vi "FRIC_navX_Internal_Serial_GenerateCommand.vi"(11 "I2C Process Loop TypeDef (in)":T1={"State Array"=[enum."INI", enum."Open"], "error"={"status"=FALSE, "code"=0, "source"=""}, "FPGA Cluster"={"Last Valid FPGA Time"=0.0, "Error Count"=0, "Initialized"=FALSE}, "Device Info"={"Interface"={"Protocol"=enum."SERIAL", "Update Rate (4Hz-100Hz)"=4, "navX Open TypeDef"=variant}, "Notify Packet"=refnum, "Loop VI Refnum"=refnum, "Ready to Close Occurrence Refnum"=refnum, "Name"=""}, "I2CDevRef"={"DevStatus"={"status"=FALSE, "code"=0, "source"=""}, "Controller"=enum."Controller 1", "Device Address"=0, "Handle"=0, "I2C Bus"=enum."Invalid"}, "Registry"=[], "Command Array"=[214, 32], "Connected?"=FALSE, "navX Device Memory Size"=85, "notification"={"navX Action"=enum."None", "Data"=variant}, "Memory Size Set"=FALSE, "SPIDevRef"={"DevStatus"={"status"=FALSE, "code"=0, "source"=""}, "Handle"=0, "Controller"=enum."Controller 1", "SPI Bus"=enum."SPI On-Board, CS0"}, "navX Serial Open"={"Serial Port"=enum."Onboard RS-232", "Stream Type"=enum."YRPH"}, "SerialPortRef"={"DevStatus"={"status"=FALSE, "code"=0, "source"=""}, "Serial Port Name"=""}, "Serial Read Buffer"="", "Serial Write Buffer"=[], "Device Number"=enum."Dev0"} {"navX Device Memory Size" format="%x"; "Command Array" items=["UNDEFINED"=0, "NAVX_INTEGRATION_CTL_RESET_VEL_X"=1, "NAVX_INTEGRATION_CTL_RESET_VEL_Y"=2, "NAVX_INTEGRATION_CTL_RESET_VEL_Z"=4, "NAVX_INTEGRATION_CTL_RESET_DISP_X"=8, "NAVX_INTEGRATION_CTL_RESET_DISP_Y"=16, "NAVX_INTEGRATION_CTL_RESET_DISP_Z"=32, "NAVX_INTEGRATION_CTL_RESET_YAW"=128]; "I2CDevRef"."Device Address" format="%.0x"; "Device Info"."Interface"."Update Rate (4Hz-100Hz)" min=4 max=60 step=1}) -> (3 "I2C Process Loop TypeDef (out)":T1={"State Array"=[enum."INI", enum."Open"], "error"={"status"=FALSE, "code"=0, "source"=""}, "FPGA Cluster"={"Last Valid FPGA Time"=0.0, "Error Count"=0, "Initialized"=FALSE}, "Device Info"={"Interface"={"Protocol"=enum."SERIAL", "Update Rate (4Hz-100Hz)"=4, "navX Open TypeDef"=variant}, "Notify Packet"=refnum, "Loop VI Refnum"=refnum, "Ready to Close Occurrence Refnum"=refnum, "Name"=""}, "I2CDevRef"={"DevStatus"={"status"=FALSE, "code"=0, "source"=""}, "Controller"=enum."Controller 1", "Device Address"=0, "Handle"=0, "I2C Bus"=enum."Invalid"}, "Registry"=[], "Command Array"=[], "Connected?"=FALSE, "navX Device Memory Size"=85, "notification"={"navX Action"=enum."None", "Data"=variant}, "Memory Size Set"=FALSE, "SPIDevRef"={"DevStatus"={"status"=FALSE, "code"=0, "source"=""}, "Handle"=0, "Controller"=enum."Controller 1", "SPI Bus"=enum."SPI On-Board, CS0"}, "navX Serial Open"={"Serial Port"=enum."Onboard RS-232", "Stream Type"=enum."YRPH"}, "SerialPortRef"={"DevStatus"={"status"=FALSE, "code"=0, "source"=""}, "Serial Port Name"=""}, "Serial Read Buffer"="", "Serial Write Buffer"=[], "Device Number"=enum."Dev0"} {"navX Device Memory Size" format="%x"; "Command Array" items=["UNDEFINED"=0, "NAVX_INTEGRATION_CTL_RESET_VEL_X"=1, "NAVX_INTEGRATION_CTL_RESET_VEL_Y"=2, "NAVX_INTEGRATION_CTL_RESET_VEL_Z"=4, "NAVX_INTEGRATION_CTL_RESET_DISP_X"=8, "NAVX_INTEGRATION_CTL_RESET_DISP_Y"=16, "NAVX_INTEGRATION_CTL_RESET_DISP_Z"=32, "NAVX_INTEGRATION_CTL_RESET_YAW"=128]; "I2CDevRef"."Device Address" format="%.0x"; "Device Info"."Interface"."Update Rate (4Hz-100Hz)" min=4 max=60 step=1})   [LabVIEW 2015, in "Untitled Library 1.lvlib"]
uses:
  Desktop/Untitled Library 1.lvlib
  TypeDefs/FRIC_navX_I2C Process Loop TypeDef.ctl
  TypeDefs/FRIC_navX_ProcessingLoopStatesTypeDef_I2C.ctl
  navX Library v2/_TypeDefs/Z900_navX_DeviceTypeDef.ctl
  navX Library v2/_TypeDefs/Z900_navX_ProtocolTypeDef.ctl
  navX Library v2/_TypeDefs/Z900_navX_NotifyPacketTypeDef.ctl
  navX Library v2/_TypeDefs/Z900_navX_ActionTypeDef.ctl
  <vilib>/Rock Robotics/SystemInterfaces/Typedef/FPGA_TypedefDigitalModule.ctl
  <vilib>/Rock Robotics/SystemInterfaces/i2clib/i2c_bus.ctl
  navX Library v2/_TypeDefs/Z900_navX_IntegrationControlRegisters.ctl
  <vilib>/Rock Robotics/WPI/SPI/WPI_SPIDevRef.ctl
  <vilib>/Rock Robotics/SystemInterfaces/spilib/spi_bus.ctl
  _NI WPI Serial USB/WPI_SerialPort_USB.ctl
  navX Library v2/_TypeDefs/Z900_navX_SerialStreamTypeDef.ctl
  <vilib>/Rock Robotics/WPI/SerialPort/WPI_SerialPortRef.ctl
  TypeDefs/FRIC_navX_DeviceNumbersTypeDef.ctl
  navX Library v2/_TypeDefs/Z900_navX_DeviceRegisters.ctl
  navX Library v2/_TypeDefs/navX Open TypeDefs/Z900_navX_OpenTypeDef_Serial.ctl
  navX Library v2/_TypeDefs/Flags/Z900_navX_Flags_CapabilityTypeDef.ctl
  navX Library v2/_TypeDefs/Z900_navX_ZeroVectorTypeDef.ctl
  navX AE v1.lvlib
  navX Library v2/navX Library v2.lvlib
  _NI WPI Serial USB/_NI WPI Serial USB.lvlib
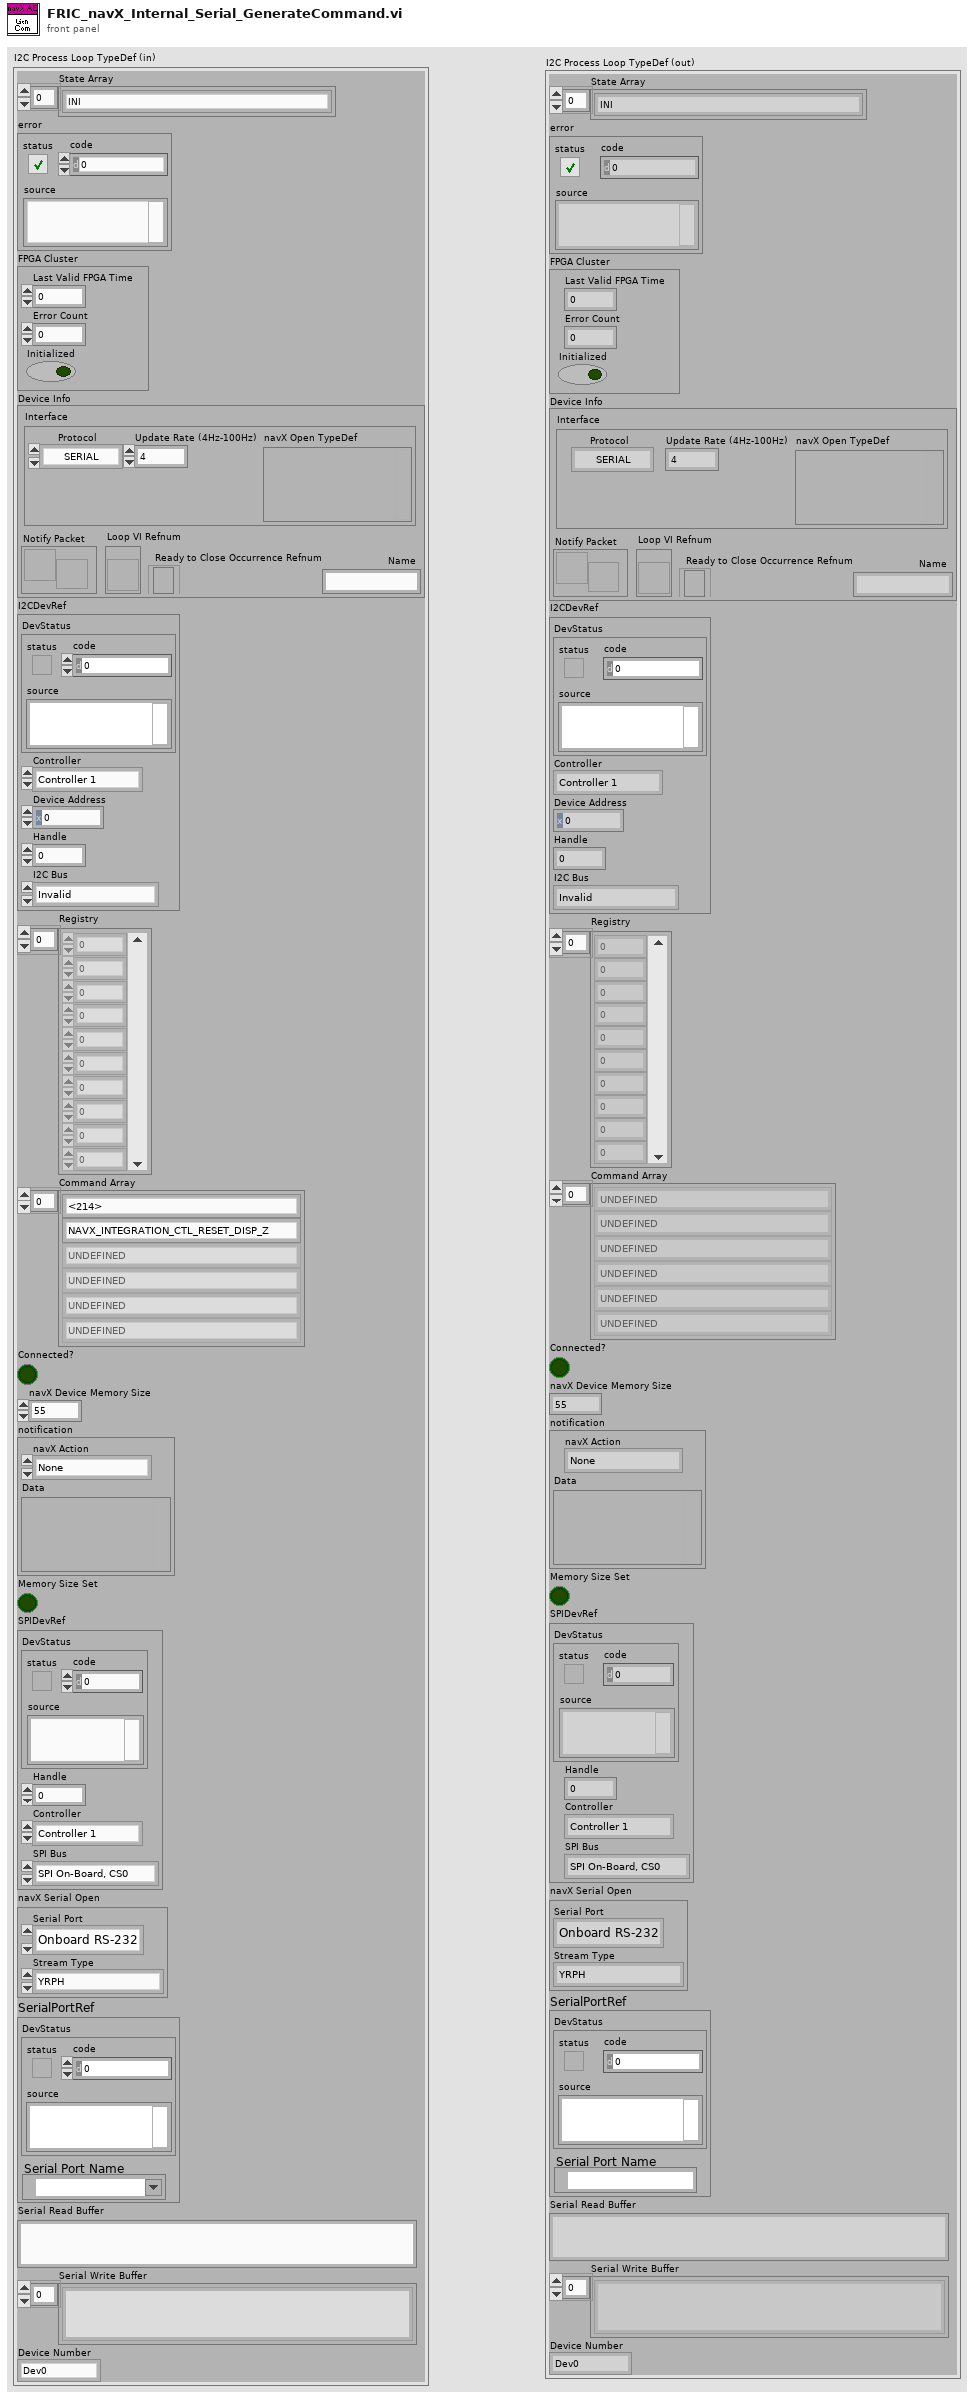
[diagram p1: front panel]
types:
  T1 = typedef "FRIC_navX_I2C Process Loop TypeDef.ctl" = cluster{"State Array":T2[], "error":errorcluster, "FPGA Cluster":cluster{"Last Valid FPGA Time":dbl, "Error Count":i32, "Initialized":bool}, "Device Info":T3, "I2CDevRef":cluster{"DevStatus":errorcluster, "Controller":T5, "Device Address":u8, "Handle":i32, "I2C Bus":T6}, "Registry":u8[], "Command Array":T7[], "Connected?":bool, "navX Device Memory Size":i32, "notification":T8, "Memory Size Set":bool, "SPIDevRef":T10, "navX Serial Open":cluster{"Serial Port":T12, "Stream Type":T13}, "SerialPortRef":T14, "Serial Read Buffer":string, "Serial Write Buffer":string[], "Device Number":T15}
  T2 = typedef "navX AE v1.lvlib/FRIC_navX_ProcessingLoopStatesTypeDef_I2C.ctl" = enum16{"Process", "INI", "Check Packets Valid", "Close", "Flush Serial", "Generate Command", "Last Packet Valid", "Open", "Read", "Reset Serial", "Set Termination Char", "Wait", "Write", "Exit"}
  T3 = typedef "navX Library v2.lvlib/Z900_navX_DeviceTypeDef.ctl" = cluster{"Interface":cluster{"Protocol":T4, "Update Rate (4Hz-100Hz)":u8, "navX Open TypeDef":variant}, "Notify Packet":refnum<notifier>, "Loop VI Refnum":refnum<vi>, "Ready to Close Occurrence Refnum":refnum<k4>, "Name":string}
  T4 = typedef "navX Library v2.lvlib/Z900_navX_ProtocolTypeDef.ctl" = enum16{"SERIAL", "I2C", "SPI"}
  T5 = typedef "FPGA_TypedefDigitalModule.ctl" = enum16{"Controller 1"}
  T6 = typedef "i2c_bus.ctl" = enum16{"I2C On-Board", "I2C MXP", "Invalid"}
  T7 = typedef "navX Library v2.lvlib/Z900_navX_IntegrationControlRegisters.ctl" = u8
  T8 = typedef "navX Library v2.lvlib/Z900_navX_NotifyPacketTypeDef.ctl" = cluster{"navX Action":T9, "Data":variant}
  T9 = typedef "navX Library v2.lvlib/Z900_navX_ActionTypeDef.ctl" = enum16{"None", "Halt", "Normal Read", "Update Serial Protocol", "Update Rate Htz", "Zero-Yaw", "Zero-Displacement", "Zero-Velocity"}
  T10 = typedef "WPI_SPIDevRef.ctl" = cluster{"DevStatus":errorcluster, "Handle":i32, "Controller":T5, "SPI Bus":T11}
  T11 = typedef "spi_bus.ctl" = enum16{"SPI On-Board, CS0", "SPI On-Board, CS1", "SPI On-Board, CS2", "SPI On-Board, CS3", "SPI MXP", "Invalid"}
  T12 = typedef "_NI WPI Serial USB.lvlib/WPI_SerialPort_USB.ctl" = enum16{"Onboard RS-232", "MXP TTL", "USB"}
  T13 = typedef "navX Library v2.lvlib/Z900_navX_SerialStreamTypeDef.ctl" = enum16{"YRPH", "Quaterinons", "Gyro/Raw", "AHRS", "AHRSAndPositioning"}
  T14 = typedef "WPI_SerialPortRef.ctl" = cluster{"DevStatus":errorcluster, "Serial Port Name":refnum<visa-resource-name>}
  T15 = typedef "Untitled Library 1.lvlib/FRIC_navX_DeviceNumbersTypeDef.ctl" = enum16{"Dev0", "Dev1", "Dev2", "Dev3", "Dev4", "Dev5", "Dev6", "Dev7", "Dev8", "Dev9", "Dev10"}
  T16 = typedef "navX Library v2.lvlib/Z900_navX_DeviceRegisters.ctl" = u8
  T17 = typedef "navX Library v2.lvlib/Z900_navX_OpenTypeDef_Serial.ctl" = cluster{"Serial Port":T12, "Stream Type":T13}
  T18 = typedef "navX Library v2.lvlib/Z900_navX_ZeroVectorTypeDef.ctl" = cluster{"X":bool, "Y":bool, "Z":bool}
  T19 = typedef "navX Library v2.lvlib/Z900_navX_Flags_CapabilityTypeDef.ctl" = u16
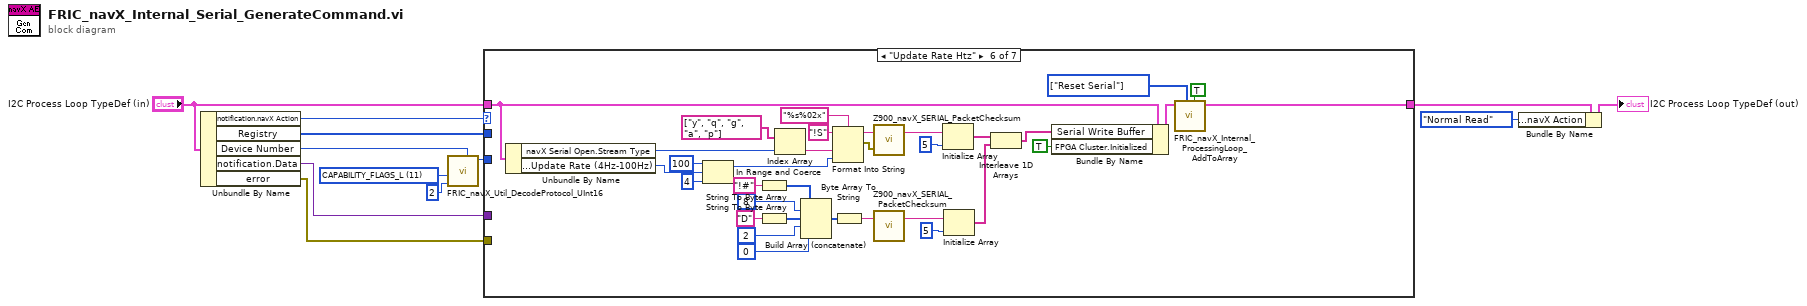
[diagram p0: block diagram]
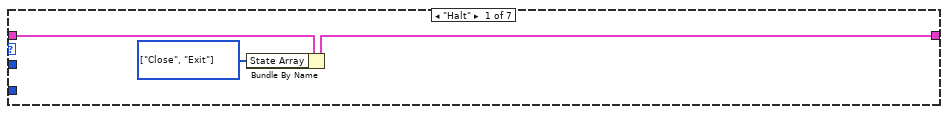
[diagram p2: hidden frame]
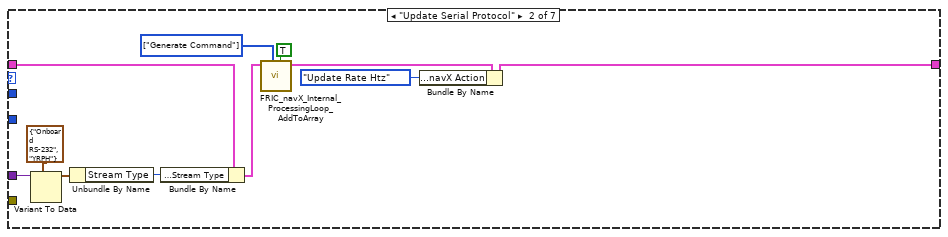
[diagram p3: hidden frame]
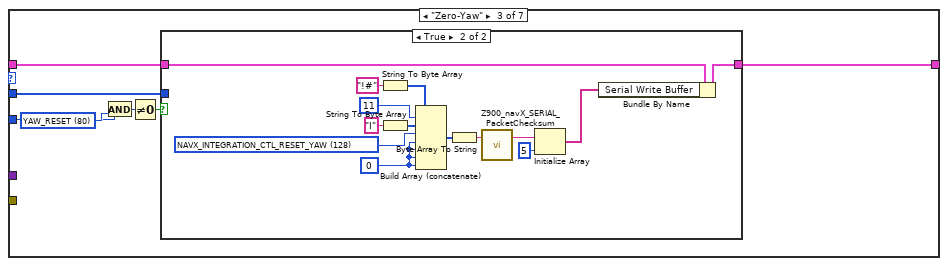
[diagram p4: hidden frame]
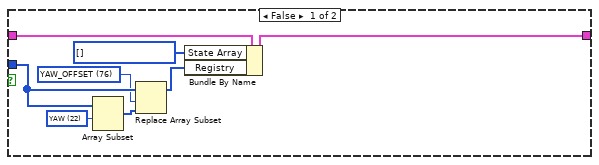
[diagram p5: hidden frame]
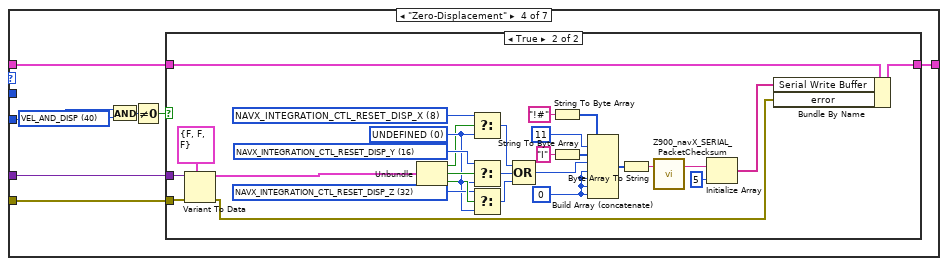
[diagram p6: hidden frame]
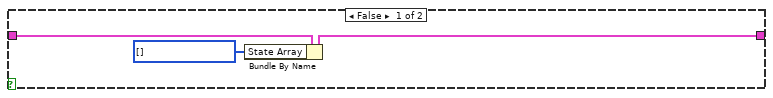
[diagram p7: hidden frame]
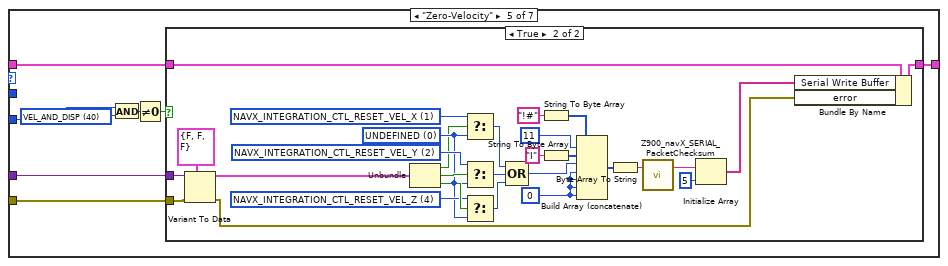
[diagram p8: hidden frame]
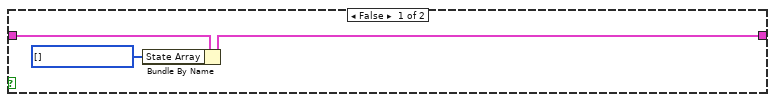
[diagram p9: hidden frame]
diagram:
  w7 = T16 11 items=["WHOAMI"=0, "HW_REV"=1, "FW_VER_MAJOR"=2, "FW_VER_MINOR"=3, "UPDATE_RATE_HZ"=4, "ACCEL_FSR_G"=5, "GYRO_FSR_DPS"=6, "OP_STATUS"=8, "CAL_STATUS"=9, "SELFTEST_STATUS"=10, "CAPABILITY_FLAGS_L"=11, "CAPABILITY_FLAGS_H"=12, "SENSOR_STATUS"=16, "TIMESTAMP"=18, "YAW"=22, "ROLL"=24, "PITCH"=26, "HEADING"=28, "FUSED_HEADING"=30, "ALTITUDE_I"=32, "ALTITUDE_D"=34, "LINERA_ACC_X"=36, "LINERA_ACC_Y"=38, "LINERA_ACC_Z"=40, "QUAT_W"=42, "QUAT_X"=44, "QUAT_Y"=46, "QUAT_Z"=48, "MPU_TEMP_C"=50, "GYRO_X"=52, "GYRO_Y"=54, "GYRO_Z"=56, "ACC_X"=58, "ACC_Y"=60, "ACC_Z"=62, "MAG_X"=64, "MAG_Y"=66, "MAG_Z"=68, "PRESSURE_I"=70, "PRESSURE_D"=72, "PRESSURE_TEMP"=74, "YAW_OFFSET"=76, "QUAT_OFFSET_W"=78, "QUAT_OFFSET_X"=80, "QUAT_OFFSET_Y"=82, "QUAT_OFFSET_Z"=84, "INTEGRATION_CONTROL"=86, "VELOCITY_X"=88, "VELOCITY_Y"=92, "VELOCITY_Z"=96, "DISPLACMENT_X"=100, "DISPLACMENT_Y"=104, "DISPLACEMENT_Z"=108] ("Device Register")
  n1 = Unbundle By Name("I2C Process Loop TypeDef (in)") -> ("notification.navX Action"=w11:T9, "Registry"=w8:u8[], "Device Number"=w1:T15, "notification.Data"=w10:variant, "error"=w9:errorcluster)
  n2 = call "FRIC_navX_Util_DecodeProtocol_UInt16.vi"("Device Number"=w1, "length"=2, "Device Register"=w7) -> ("Value"=w5:u16)  [unwired: 8 in]
  n3 = case shown="\"Update Rate Htz\"" w11 {
    tunnel: "I2C Process Loop TypeDef (in)" -> [w15 w22 w29 w61 w101 w168 w169]
    tunnel: [w14 w18 w28 w62 w102 w144 w169] -> w3
    tunnel: w10 -> [_ w26 _ w63 w103 _ _]
    tunnel: w9 -> [_ _ _ w60 w100 _ _]
    tunnel: w8 -> [_ _ w30 _ _ _ _]
    tunnel: w5 -> [_ _ w27 w57 w97 _ _]
    frame "Halt" {
      w13 = T2[] [enum."Close", enum."Exit"] items=["Process", "INI", "Check Packets Valid", "Close", "Flush Serial", "Generate Command", "Last Packet Valid", "Open", "Read", "Reset Serial", "Set Termination Char", "Wait", "Write", "Exit"]
      n4 = Bundle By Name(cluster=w15, "State Array"=w13) -> (w14:T1)
    }
    frame "Update Serial Protocol" {
      w20 = T2[] [enum."Generate Command"] items=["Process", "INI", "Check Packets Valid", "Close", "Flush Serial", "Generate Command", "Last Packet Valid", "Open", "Read", "Reset Serial", "Set Termination Char", "Wait", "Write", "Exit"] ("States Array")
      n5 = Variant To Data(type=T17 {"Serial Port"=enum."Onboard RS-232", "Stream Type"=enum."YRPH"} ("navX Serial Open"), Variant=w26) -> (data=w24:T17)  [unwired: 1 in, 1 out]
      n6 = Unbundle By Name(w24) -> ("Stream Type"=w23:T13)
      n7 = Bundle By Name(cluster=w22, "navX Serial Open.Stream Type"=w23) -> (w21:T1)
      n8 = call "FRIC_navX_Internal_ProcessingLoop_AddToArray.vi"("Add to beginning"=TRUE, "States Array"=w20, "I2C Process Loop TypeDef (in)"=w21) -> ("I2C Process Loop TypeDef (out)"=w19:T1)  [unwired: 8 in]
      n9 = Bundle By Name(cluster=w19, "notification.navX Action"=Z900_navX_ActionTypeDef."Update Rate Htz") -> (w18:T1)
    }
    frame "Zero-Yaw" {
      w32 = T19 80 items=["OMNIMOUNT"=4, "OMNIMOUNT_CONFIG_MASK"=38, "VEL_AND_DISP"=40, "YAW_RESET"=80] ("Capability Flag")
      n10 = And(x=w27, y=w32) -> (x .and. y?=w33:T19)
      n11 = Not Equal To 0?(x=w33) -> (x != 0?=w31:bool)
      n12 = case shown="True" w31 {
        tunnel: w30 -> [w41 _]
        tunnel: w29 -> [w37 w44]
        tunnel: [w36 w43] -> w28
        frame False {
          w35 = T2[] [] items=["Process", "INI", "Check Packets Valid", "Close", "Flush Serial", "Generate Command", "Last Packet Valid", "Open", "Read", "Reset Serial", "Set Termination Char", "Wait", "Write", "Exit"] ("State Array")
          w38 = T16 76 items=["WHOAMI"=0, "HW_REV"=1, "FW_VER_MAJOR"=2, "FW_VER_MINOR"=3, "UPDATE_RATE_HZ"=4, "ACCEL_FSR_G"=5, "GYRO_FSR_DPS"=6, "OP_STATUS"=8, "CAL_STATUS"=9, "SELFTEST_STATUS"=10, "CAPABILITY_FLAGS_L"=11, "CAPABILITY_FLAGS_H"=12, "SENSOR_STATUS"=16, "TIMESTAMP"=18, "YAW"=22, "ROLL"=24, "PITCH"=26, "HEADING"=28, "FUSED_HEADING"=30, "ALTITUDE_I"=32, "ALTITUDE_D"=34, "LINERA_ACC_X"=36, "LINERA_ACC_Y"=38, "LINERA_ACC_Z"=40, "QUAT_W"=42, "QUAT_X"=44, "QUAT_Y"=46, "QUAT_Z"=48, "MPU_TEMP_C"=50, "GYRO_X"=52, "GYRO_Y"=54, "GYRO_Z"=56, "ACC_X"=58, "ACC_Y"=60, "ACC_Z"=62, "MAG_X"=64, "MAG_Y"=66, "MAG_Z"=68, "PRESSURE_I"=70, "PRESSURE_D"=72, "PRESSURE_TEMP"=74, "YAW_OFFSET"=76, "QUAT_OFFSET_W"=78, "QUAT_OFFSET_X"=80, "QUAT_OFFSET_Y"=82, "QUAT_OFFSET_Z"=84, "INTEGRATION_CONTROL"=86, "VELOCITY_X"=88, "VELOCITY_Y"=92, "VELOCITY_Z"=96, "DISPLACMENT_X"=100, "DISPLACMENT_Y"=104, "DISPLACEMENT_Z"=108] ("Device Register")
          w39 = T16 22 items=["WHOAMI"=0, "HW_REV"=1, "FW_VER_MAJOR"=2, "FW_VER_MINOR"=3, "UPDATE_RATE_HZ"=4, "ACCEL_FSR_G"=5, "GYRO_FSR_DPS"=6, "OP_STATUS"=8, "CAL_STATUS"=9, "SELFTEST_STATUS"=10, "CAPABILITY_FLAGS_L"=11, "CAPABILITY_FLAGS_H"=12, "SENSOR_STATUS"=16, "TIMESTAMP"=18, "YAW"=22, "ROLL"=24, "PITCH"=26, "HEADING"=28, "FUSED_HEADING"=30, "ALTITUDE_I"=32, "ALTITUDE_D"=34, "LINERA_ACC_X"=36, "LINERA_ACC_Y"=38, "LINERA_ACC_Z"=40, "QUAT_W"=42, "QUAT_X"=44, "QUAT_Y"=46, "QUAT_Z"=48, "MPU_TEMP_C"=50, "GYRO_X"=52, "GYRO_Y"=54, "GYRO_Z"=56, "ACC_X"=58, "ACC_Y"=60, "ACC_Z"=62, "MAG_X"=64, "MAG_Y"=66, "MAG_Z"=68, "PRESSURE_I"=70, "PRESSURE_D"=72, "PRESSURE_TEMP"=74, "YAW_OFFSET"=76, "QUAT_OFFSET_W"=78, "QUAT_OFFSET_X"=80, "QUAT_OFFSET_Y"=82, "QUAT_OFFSET_Z"=84, "INTEGRATION_CONTROL"=86, "VELOCITY_X"=88, "VELOCITY_Y"=92, "VELOCITY_Z"=96, "DISPLACMENT_X"=100, "DISPLACMENT_Y"=104, "DISPLACEMENT_Z"=108] ("Device Register")
          n13 = Array Subset(array=w41, index=w39) -> (w40:u8[])  [unwired: 1 in]
          n14 = Replace Array Subset(array=w41, new element=w40, index=w38) -> (w34:u8[])
          n15 = Bundle By Name(cluster=w37, "State Array"=w35, "Registry"=w34) -> (w36:T1)
        }
        frame True {
          w53 = 0
          w47 = T7 128 items=["UNDEFINED"=0, "NAVX_INTEGRATION_CTL_RESET_VEL_X"=1, "NAVX_INTEGRATION_CTL_RESET_VEL_Y"=2, "NAVX_INTEGRATION_CTL_RESET_VEL_Z"=4, "NAVX_INTEGRATION_CTL_RESET_DISP_X"=8, "NAVX_INTEGRATION_CTL_RESET_DISP_Y"=16, "NAVX_INTEGRATION_CTL_RESET_DISP_Z"=32, "NAVX_INTEGRATION_CTL_RESET_YAW"=128] ("Integration Control Register")
          n16 = String To Byte Array(string="!#" ("initial string")) -> (unsigned byte array=w48:u8[])
          n17 = String To Byte Array(string="I" ("initial string")) -> (unsigned byte array=w50:u8[])
          n18 = Build Array (concatenate)(w48, 11, w50, w47, w53, w53, w53, w53) -> (w49:i32[])
          n19 = Byte Array To String(unsigned byte array=w49) -> (string=w45:string)
          n20 = call "Z900_navX_SERIAL_PacketChecksum.vi"("Packet"=w45) -> ("Terminated Packet"=w54:string)  [unwired: 1 in, 1 out]
          n21 = Initialize Array(w54, 5 ("dimension size")) -> (w42:string[])
          n22 = Bundle By Name(cluster=w44, "Serial Write Buffer"=w42) -> (w43:T1)
        }
      }
    }
    frame "Zero-Displacement" {
      w59 = T19 40 items=["OMNIMOUNT"=4, "OMNIMOUNT_CONFIG_MASK"=38, "VEL_AND_DISP"=40, "YAW_RESET"=80] ("Capability Flag")
      n23 = And(x=w57, y=w59) -> (x .and. y?=w58:T19)
      n24 = Not Equal To 0?(x=w58) -> (x != 0?=w56:bool)
      n25 = case shown="True" w56 {
        tunnel: w63 -> [_ w83]
        tunnel: [w65 w82] -> w62
        tunnel: w61 -> [w66 w80]
        tunnel: w60 -> [_ w79]
        frame False {
          w64 = T2[] [] items=["Process", "INI", "Check Packets Valid", "Close", "Flush Serial", "Generate Command", "Last Packet Valid", "Open", "Read", "Reset Serial", "Set Termination Char", "Wait", "Write", "Exit"] ("State Array")
          n26 = Bundle By Name(cluster=w66, "State Array"=w64) -> (w65:T1)
        }
        frame True {
          w76 = 0
          w87 = T7 0 items=["UNDEFINED"=0, "NAVX_INTEGRATION_CTL_RESET_VEL_X"=1, "NAVX_INTEGRATION_CTL_RESET_VEL_Y"=2, "NAVX_INTEGRATION_CTL_RESET_VEL_Z"=4, "NAVX_INTEGRATION_CTL_RESET_DISP_X"=8, "NAVX_INTEGRATION_CTL_RESET_DISP_Y"=16, "NAVX_INTEGRATION_CTL_RESET_DISP_Z"=32, "NAVX_INTEGRATION_CTL_RESET_YAW"=128] ("f")
          w88 = T7 32 items=["UNDEFINED"=0, "NAVX_INTEGRATION_CTL_RESET_VEL_X"=1, "NAVX_INTEGRATION_CTL_RESET_VEL_Y"=2, "NAVX_INTEGRATION_CTL_RESET_VEL_Z"=4, "NAVX_INTEGRATION_CTL_RESET_DISP_X"=8, "NAVX_INTEGRATION_CTL_RESET_DISP_Y"=16, "NAVX_INTEGRATION_CTL_RESET_DISP_Z"=32, "NAVX_INTEGRATION_CTL_RESET_YAW"=128] ("Integration Control Register")
          w89 = T7 16 items=["UNDEFINED"=0, "NAVX_INTEGRATION_CTL_RESET_VEL_X"=1, "NAVX_INTEGRATION_CTL_RESET_VEL_Y"=2, "NAVX_INTEGRATION_CTL_RESET_VEL_Z"=4, "NAVX_INTEGRATION_CTL_RESET_DISP_X"=8, "NAVX_INTEGRATION_CTL_RESET_DISP_Y"=16, "NAVX_INTEGRATION_CTL_RESET_DISP_Z"=32, "NAVX_INTEGRATION_CTL_RESET_YAW"=128] ("Integration Control Register")
          w86 = T7 8 items=["UNDEFINED"=0, "NAVX_INTEGRATION_CTL_RESET_VEL_X"=1, "NAVX_INTEGRATION_CTL_RESET_VEL_Y"=2, "NAVX_INTEGRATION_CTL_RESET_VEL_Z"=4, "NAVX_INTEGRATION_CTL_RESET_DISP_X"=8, "NAVX_INTEGRATION_CTL_RESET_DISP_Y"=16, "NAVX_INTEGRATION_CTL_RESET_DISP_Z"=32, "NAVX_INTEGRATION_CTL_RESET_YAW"=128] ("Integration Control Register")
          n27 = Variant To Data(error in=w79, type=T18 {"X"=FALSE, "Y"=FALSE, "Z"=FALSE} ("Zero Vector"), Variant=w83) -> (data=w84:T18, error out=w81:errorcluster)
          n28 = Unbundle(w84) -> ("X"=w85:bool, "Y"=w90:bool, "Z"=w91:bool)
          n29 = Select(t=w86, s=w85, f=w87) -> (s? t:f=w92:T7)
          n30 = Select(t=w89, s=w90, f=w87) -> (s? t:f=w93:T7)
          n31 = Select(t=w88, s=w91, f=w87) -> (s? t:f=w94:T7)
          n32 = Compound Arithmetic op=OR(w92, w93, w94) -> (w68:T7)
          n33 = String To Byte Array(string="!#" ("initial string")) -> (unsigned byte array=w71:u8[])
          n34 = String To Byte Array(string="I" ("initial string")) -> (unsigned byte array=w73:u8[])
          n35 = Build Array (concatenate)(w71, 11, w73, w68, w76, w76, w76, w76) -> (w72:i32[])
          n36 = Byte Array To String(unsigned byte array=w72) -> (string=w69:string)
          n37 = call "Z900_navX_SERIAL_PacketChecksum.vi"("Packet"=w69) -> ("Terminated Packet"=w77:string)  [unwired: 1 in, 1 out]
          n38 = Initialize Array(w77, 5 ("dimension size")) -> (w67:string[])
          n39 = Bundle By Name(cluster=w80, "Serial Write Buffer"=w67, "error"=w81) -> (w82:T1)
        }
      }
    }
    frame "Zero-Velocity" {
      w99 = T19 40 items=["OMNIMOUNT"=4, "OMNIMOUNT_CONFIG_MASK"=38, "VEL_AND_DISP"=40, "YAW_RESET"=80] ("Capability Flag")
      n40 = And(x=w97, y=w99) -> (x .and. y?=w98:T19)
      n41 = Not Equal To 0?(x=w98) -> (x != 0?=w96:bool)
      n42 = case shown="True" w96 {
        tunnel: w103 -> [_ w123]
        tunnel: [w104 w122] -> w102
        tunnel: w101 -> [w105 w120]
        tunnel: w100 -> [_ w119]
        frame False {
          w106 = T2[] [] items=["Process", "INI", "Check Packets Valid", "Close", "Flush Serial", "Generate Command", "Last Packet Valid", "Open", "Read", "Reset Serial", "Set Termination Char", "Wait", "Write", "Exit"] ("State Array")
          n43 = Bundle By Name(cluster=w105, "State Array"=w106) -> (w104:T1)
        }
        frame True {
          w116 = 0
          w128 = T7 0 items=["UNDEFINED"=0, "NAVX_INTEGRATION_CTL_RESET_VEL_X"=1, "NAVX_INTEGRATION_CTL_RESET_VEL_Y"=2, "NAVX_INTEGRATION_CTL_RESET_VEL_Z"=4, "NAVX_INTEGRATION_CTL_RESET_DISP_X"=8, "NAVX_INTEGRATION_CTL_RESET_DISP_Y"=16, "NAVX_INTEGRATION_CTL_RESET_DISP_Z"=32, "NAVX_INTEGRATION_CTL_RESET_YAW"=128] ("f")
          w129 = T7 4 items=["UNDEFINED"=0, "NAVX_INTEGRATION_CTL_RESET_VEL_X"=1, "NAVX_INTEGRATION_CTL_RESET_VEL_Y"=2, "NAVX_INTEGRATION_CTL_RESET_VEL_Z"=4, "NAVX_INTEGRATION_CTL_RESET_DISP_X"=8, "NAVX_INTEGRATION_CTL_RESET_DISP_Y"=16, "NAVX_INTEGRATION_CTL_RESET_DISP_Z"=32, "NAVX_INTEGRATION_CTL_RESET_YAW"=128] ("Integration Control Register")
          w130 = T7 2 items=["UNDEFINED"=0, "NAVX_INTEGRATION_CTL_RESET_VEL_X"=1, "NAVX_INTEGRATION_CTL_RESET_VEL_Y"=2, "NAVX_INTEGRATION_CTL_RESET_VEL_Z"=4, "NAVX_INTEGRATION_CTL_RESET_DISP_X"=8, "NAVX_INTEGRATION_CTL_RESET_DISP_Y"=16, "NAVX_INTEGRATION_CTL_RESET_DISP_Z"=32, "NAVX_INTEGRATION_CTL_RESET_YAW"=128] ("Integration Control Register")
          w127 = T7 1 items=["UNDEFINED"=0, "NAVX_INTEGRATION_CTL_RESET_VEL_X"=1, "NAVX_INTEGRATION_CTL_RESET_VEL_Y"=2, "NAVX_INTEGRATION_CTL_RESET_VEL_Z"=4, "NAVX_INTEGRATION_CTL_RESET_DISP_X"=8, "NAVX_INTEGRATION_CTL_RESET_DISP_Y"=16, "NAVX_INTEGRATION_CTL_RESET_DISP_Z"=32, "NAVX_INTEGRATION_CTL_RESET_YAW"=128] ("Integration Control Register")
          n44 = Variant To Data(error in=w119, type=T18 {"X"=FALSE, "Y"=FALSE, "Z"=FALSE} ("Zero Vector"), Variant=w123) -> (data=w124:T18, error out=w121:errorcluster)
          n45 = Unbundle(w124) -> ("X"=w126:bool, "Y"=w131:bool, "Z"=w132:bool)
          n46 = Select(t=w127, s=w126, f=w128) -> (s? t:f=w133:T7)
          n47 = Select(t=w130, s=w131, f=w128) -> (s? t:f=w134:T7)
          n48 = Select(t=w129, s=w132, f=w128) -> (s? t:f=w135:T7)
          n49 = Compound Arithmetic op=OR(w133, w134, w135) -> (w108:T7)
          n50 = String To Byte Array(string="!#" ("initial string")) -> (unsigned byte array=w111:u8[])
          n51 = String To Byte Array(string="I" ("initial string")) -> (unsigned byte array=w113:u8[])
          n52 = Build Array (concatenate)(w111, 11, w113, w108, w116, w116, w116, w116) -> (w112:i32[])
          n53 = Byte Array To String(unsigned byte array=w112) -> (string=w109:string)
          n54 = call "Z900_navX_SERIAL_PacketChecksum.vi"("Packet"=w109) -> ("Terminated Packet"=w117:string)  [unwired: 1 in, 1 out]
          n55 = Initialize Array(w117, 5 ("dimension size")) -> (w107:string[])
          n56 = Bundle By Name(cluster=w120, "Serial Write Buffer"=w107, "error"=w121) -> (w122:T1)
        }
      }
    }
    frame "Update Rate Htz" {
      w142 = T2[] [enum."Reset Serial"] items=["Process", "INI", "Check Packets Valid", "Close", "Flush Serial", "Generate Command", "Last Packet Valid", "Open", "Read", "Reset Serial", "Set Termination Char", "Wait", "Write", "Exit"] ("States Array")
      n57 = Unbundle By Name(w168) -> ("navX Serial Open.Stream Type"=w163:T13, "Device Info.Interface.Update Rate (4Hz-100Hz)"=w138:u8)
      n58 = In Range and Coerce(upper limit=u8 100, x=w138, lower limit=u8 4) -> (coerced(x)=w137:u8)  [unwired: 1 out]
      n59 = String To Byte Array(string="!#" ("initial string")) -> (unsigned byte array=w156:u8[])
      n60 = String To Byte Array(string="D" ("initial string")) -> (unsigned byte array=w154:u8[])
      n61 = Index Array(array=string[] ["y", "q", "g", "a", "p"], index=w163) -> (element=w164:string)
      n62 = Build Array (concatenate)(w156, 8, w154, 2, 0) -> (w151:i32[])
      n63 = Format Into String(format string="%s%02x", initial string="!S", w164, w137) -> (resulting string=w162:string, error out=w161:errorcluster)  [unwired: 1 in]
      n64 = Byte Array To String(unsigned byte array=w151) -> (string=w160:string)
      n65 = call "Z900_navX_SERIAL_PacketChecksum.vi"("error in (no error)"=w161, "Packet"=w162) -> ("Terminated Packet"=w148:string)  [unwired: 1 out]
      n66 = call "Z900_navX_SERIAL_PacketChecksum.vi"("Packet"=w160) -> ("Terminated Packet"=w150:string)  [unwired: 1 in, 1 out]
      n67 = Initialize Array(w148, 5 ("dimension size")) -> (w147:string[])
      n68 = Initialize Array(w150, 5 ("dimension size")) -> (w146:string[])
      n69 = Interleave 1D Arrays(w147, w146) -> (w145:string[])
      n70 = Bundle By Name(cluster=w168, "Serial Write Buffer"=w145, "FPGA Cluster.Initialized"=TRUE) -> (w143:T1)
      n71 = call "FRIC_navX_Internal_ProcessingLoop_AddToArray.vi"("Add to beginning"=TRUE, "States Array"=w142, "I2C Process Loop TypeDef (in)"=w143) -> ("I2C Process Loop TypeDef (out)"=w144:T1)  [unwired: 8 in]
    }
    frame "Normal Read", Default {
    }
  }
  n72 = Bundle By Name(cluster=w3, "notification.navX Action"=Z900_navX_ActionTypeDef."Normal Read") -> (→"I2C Process Loop TypeDef (out)":T1)
